vi "Report Mean Data.vi"(10 "Max Array":dbl[][](array[numeric]), 11 "Mean Array in":dbl[][](array[numeric])) -> (2 "Max Array out":i32[][](array[numeric]), 3 "Mean Array out":i32[][](array[numeric]))   [LabVIEW 2020]
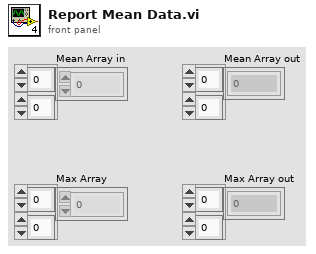
[diagram p1: front panel]
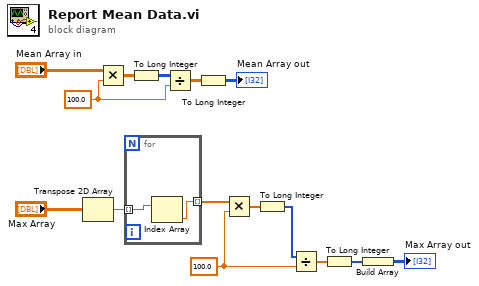
[diagram p0: block diagram]
diagram:
  w9 = 100.0 ("Numeric")
  w8 = 100.0 ("Numeric")
  n1 = Transpose 2D Array(2D array="Max Array") -> (transposed array=w2:dbl[][])
  n2 = Multiply(x="Mean Array in", y=w8) -> (x*y=w7:dbl[][])
  n3 = for {
    tunnel: w2 -> [w17] mode=indexing
    tunnel: [w16] -> w12 mode=indexing
    n4 = Index Array(array=w17) -> (element=w16:dbl)  [unwired: 1 in]
  }
  n5 = To Long Integer(number=w7) -> (32bit integer=w6:i32[][])
  n6 = Divide(x=w6, y=w8) -> (x/y=w5:dbl[][])
  n7 = To Long Integer(number=w5) -> (32bit integer=→"Mean Array out":i32[][])
  n8 = Multiply(x=w12, y=w9) -> (x*y=w10:dbl[])
  n9 = To Long Integer(number=w10) -> (32bit integer=w11:i32[])
  n10 = Divide(x=w11, y=w9) -> (x/y=w13:dbl[])
  n11 = To Long Integer(number=w13) -> (32bit integer=w14:i32[])
  n12 = Build Array(w14) -> (→"Max Array out":i32[][])
